vi "Set Out.vi"(8 "error in":errorcluster, 11 "6509 in":refnum<class "6509.lvclass">) -> (0 "error out":errorcluster, 3 "6509 out":refnum<class "6509.lvclass">)   [LabVIEW 2019, in "6509.lvlib" / "6509.lvclass"]
uses:
  Library/6509.lvclass
  C:/Users/Public/Documents/Development/builds/Instruments/DIG_IO.lvlibp/Library/DIG_IO.lvclass
  Library/6509.lvclass/6509.ctl
  <vilib>/DAQmx/write.llb/DAQmx Write (Digital 1D U8 NChan 1Samp).vi
  builds/Instruments/DIG_IO.lvlibp/Accessors/Read IO_Mode.vi
  builds/Instruments/DIG_IO.lvlibp/Accessors/Read Digital.vi
  builds/Instruments/DIG_IO.lvlibp/Accessors/Read Control.vi
  <vilib>/DAQmx/miscellaneous.llb/DAQmx Fill In Error Info.vi
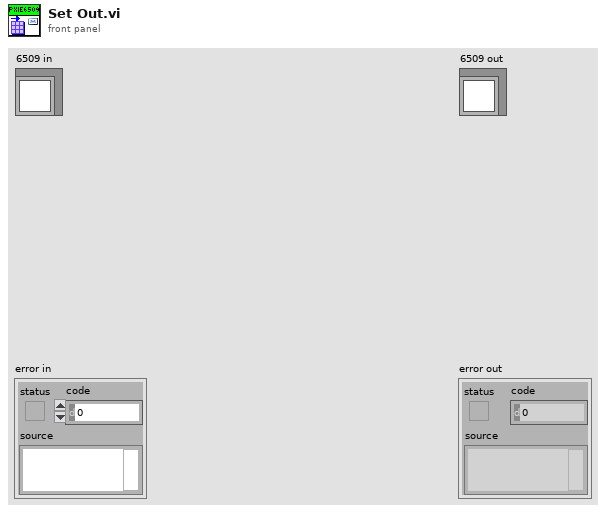
[diagram p1: front panel]
types:
  T1 = typedef "DIG_IO.lvlibp/DIG_IO.lvclass/IO Mode.ctl" = enum16{"IO", "IN", "OUT"}
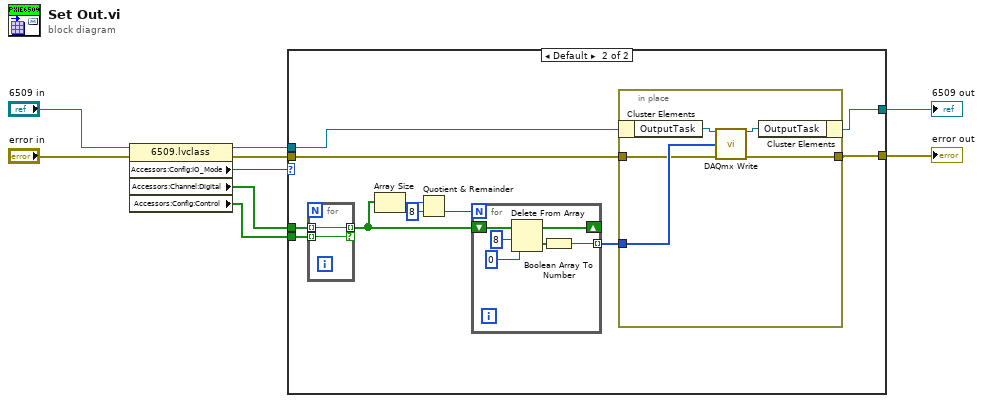
[diagram p0: block diagram]
diagram:
  n1 = property class="6509.lvclass"(reference="6509 in", error in="error in") -> (reference out=w8:refnum<class "6509.lvclass">, error out=w9:errorcluster, "Accessors:Config:IO_Mode"=w1:T1, "Accessors:Channel:Digital"=w6:bool[], "Accessors:Config:Control"=w7:bool[])
  n2 = case shown="Default" w1 {
    tunnel: w9 -> [w10 w22]
    tunnel: w8 -> [w11 w20]
    tunnel: w7 -> [_ w19]
    tunnel: w6 -> [_ w18]
    tunnel: [w10 w17] -> w3
    tunnel: [w11 w16] -> w2
    frame "IN" {
    }
    frame Default {
      n3 = for {
        tunnel: w18 -> [w35] mode=indexing
        tunnel: w19 -> [w34] mode=indexing
        tunnel: [w35] -> w15 mode=indexing if=w34
      }
      n4 = Array Size(array=w15) -> (size(s)=w14:i32)
      n5 = Quotient & Remainder(x=w14, y=8) -> (floor(x/y)=w12:i32)  [unwired: 1 out]
      n6 = for {
        N: w12 -> [_]
        shift-right: [w32] -> _
        shift-left: w15 -> [w33]
        tunnel: [w28] -> w21 mode=indexing
        n7 = Delete From Array(array=w33, length=8, index=0) -> (deleted portion=w29:bool[], array with subset deleted=w32:bool[])
        n8 = Boolean Array To Number(Boolean array=w29) -> (number=w28:u8)
      }
      n9 = in-place {
        in-place-border: w21 -> [w25]
        in-place-border: w22 -> [w24]
        in-place-border: [w23] -> w17
        n10 = in-place-cluster #1(w20) -> ("OutputTask"=w27:refnum<k21>)
        n11 = call-poly <vilib>:"DAQmx Write.vi"("task/channels in"=w27, "data"=w25, "error in"=w24) -> ("task out"=w26:refnum<k21>, "error out"=w23:errorcluster)  [unwired: 10 in, 1 out]
        n12 = in-place-cluster #1("OutputTask"=w26) -> (w16:refnum<class "6509.lvclass">)
      }
    }
  }
  "error out" <- w3
  "6509 out" <- w2
